vi "Initialize-object-wrapper-example.vi"(8 "error in (no error)":errorcluster, 10 "Main vi ref.":refnum<vi>) -> (0 "error out":errorcluster, 3 "Reference out":T1)   [LabVIEW 2013, in "PaneToggle.lvlib" / "Panes.lvclass"]
uses:
  Panes.lvclass
  Object-reference.ctl
  Pane-settings.ctl
  Pane-names.ctl
  Splitter-settings.ctl
  Splitter-names.ctl
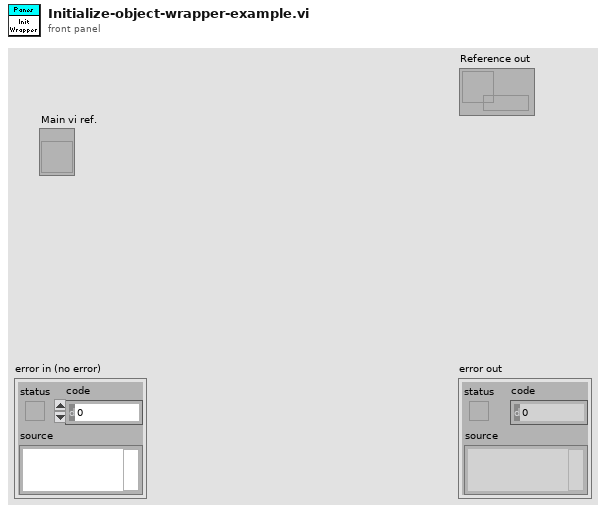
[diagram p1: front panel]
types:
  T1 = typedef "PaneToggle.lvlib/Panes.lvclass/Object-reference.ctl" = refnum<data-value>
  T2 = typedef "PaneToggle.lvlib/Panes.lvclass/Pane-settings.ctl" = cluster{"Pane-name":T3, "Startup visible?":bool, "Currently visible?":bool, "Splitters":T4[], "Pane-reference":refnum<vi>}
  T3 = typedef "PaneToggle.lvlib/Panes.lvclass/Pane-names.ctl" = enum16{"Toolbar", "Help bar", "Toolbar lower border", "Main panel", "Status bar upper border", "General state bar", "Information bar"}
  T4 = typedef "PaneToggle.lvlib/Panes.lvclass/Splitter-settings.ctl" = cluster{"Splitter-name":T5, "Position shown":i32, "Position hidden":i32, "Splitter reference":refnum<vi>}
  T5 = typedef "PaneToggle.lvlib/Panes.lvclass/Splitter-names.ctl" = enum16{"Upper toolbar splitter", "Help bar splitter", "Lower toolbar splitter", "Upper status bar splitter", "Lower status bar splitter", "Left status bar splitter"}
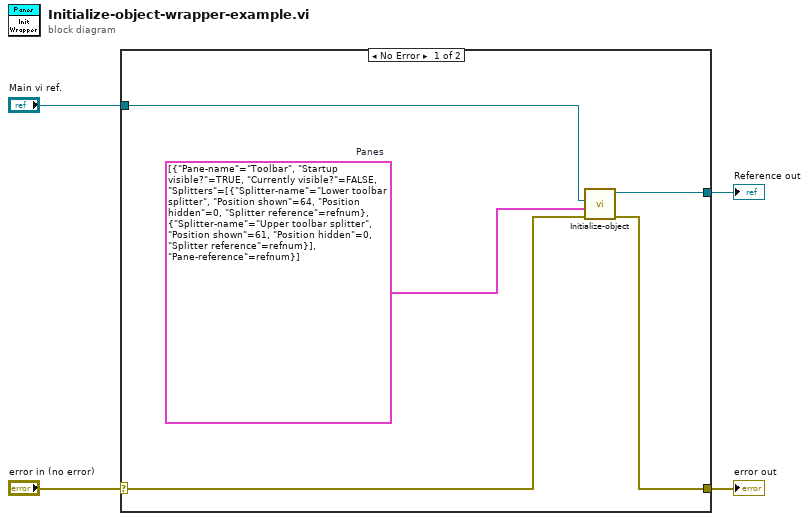
[diagram p0: block diagram]
diagram:
  n1 = case shown="No Error" "error in (no error)" {
    selector: "error in (no error)" -> [w7 w10]
    tunnel: [w8 w10] -> w3
    tunnel: [w9 _] -> w2
    tunnel: "Main vi ref." -> [w5 _]
    frame No Error {
      w6 = T2[] [{"Pane-name"=enum."Toolbar", "Startup visible?"=TRUE, "Currently visible?"=FALSE, "Splitters"=[{"Splitter-name"=enum."Lower toolbar splitter", "Position shown"=64, "Position hidden"=0, "Splitter reference"=refnum}, {"Splitter-name"=enum."Upper toolbar splitter", "Position shown"=61, "Position hidden"=0, "Splitter reference"=refnum}], "Pane-reference"=refnum}]  # Panes
      n2 = call "Initialize-object.vi"("error in (no error)"=w7, "Panes settings"=w6, "VI Reference"=w5) -> ("error out"=w8:errorcluster, "Panes out"=w9:T1)  [unwired: 7 in]
    }
    frame Error {
    }
  }
  "error out" <- w3
  "Reference out" <- w2
